vi "Add Extensions to Available Jobs.vi"(8 "error in (no error)":errorcluster) -> (0 "error out":errorcluster)   [LabVIEW 2014]
uses:
  <vilib>/Utility/traverseref.llb/TRef TravTarget.ctl
  <vilib>/Utility/miscctls.llb/LVPointTypeDef.ctl
  <vilib>/Utility/traverseref.llb/VI Scripting - Traverse.lvlib
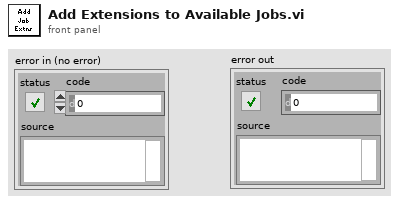
[diagram p1: front panel]
types:
  T1 = typedef "TRef TravTarget.ctl" = enum16{"FP", "BD", "Other"}
  T2 = typedef "LVPointTypeDef.ctl" = cluster{"Horizontal":i16, "Vertical":i16}
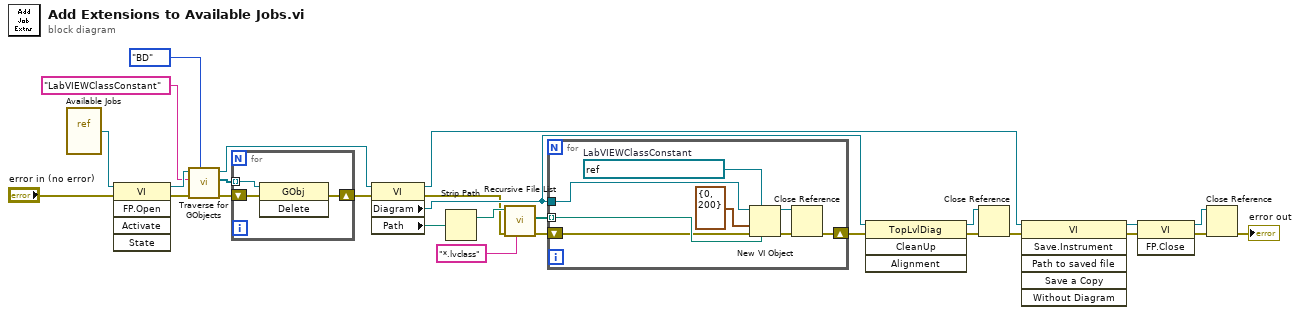
[diagram p0: block diagram]
diagram:
  n1 = vi-ref "Available Jobs.vi"() -> (w27:refnum<vi>)
  n2 = invoke class="VI" method="FP.Open"(reference=w27, error in="error in (no error)") -> (reference out=w8:refnum<vi>, error out=w6:errorcluster)  [unwired: 3 in, 3 out]
  n3 = call <vilib>:"Traverse for GObjects.vi"("Traverse Target"=TRef_TravTarget."BD", "error in (no error)"=w6, "Class Name"="LabVIEWClassConstant", "VI Refnum"=w8) -> ("error out"=w4:errorcluster, "References"=w3:refnum<vi>[], "dup VI Refnum"=w2:refnum<vi>)  [unwired: 4 in, 1 out]
  n4 = for {
    shift-right: [w28] -> w1
    shift-left: w4 -> [w29]
    tunnel: w3 -> [w30] mode=indexing
    n5 = invoke class="GObj" method="Delete"(reference=w30, error in=w29) -> (error out=w28:errorcluster)  [unwired: 1 in, 2 out]
  }
  n6 = property class="VI"(reference=w2, error in=w1) -> (reference out=w15:refnum<vi>, error out=w20:errorcluster, "Diagram"=w22:refnum<vi>, "Path"=w26:path)
  n7 = Strip Path(path=w26) -> (stripped path=w25:path)  [unwired: 1 out]
  n8 = call <vilib>:"Recursive File List.vi"("pattern"="*.lvclass", "error in (no error)"=w20, "Folder Path"=w25) -> ("error out"=w19:errorcluster, "All Files in Dir"=w23:path[])  [unwired: 4 in, 3 out]
  n9 = for {
    tunnel: w22 -> [w38]
    tunnel: w23 -> [w35] mode=indexing
    shift-right: [w31] -> w21
    shift-left: w19 -> [w34]
    w37 = refnum<vi> refnum  # LabVIEWClassConstant
    n10 = New VI Object(vi object class=w37, owner refnum=w38, position/next to=T2 {"Horizontal"=0, "Vertical"=200} ("location"), 6:w35, 8:w34) -> (object refnum=w32:refnum<vi>, 0:w33:errorcluster)  [unwired: 3 in]
    n11 = Close Reference(reference=w32, error in (no error)=w33) -> (error out=w31:errorcluster)
  }
  n12 = invoke class="TopLvlDiag" method="CleanUp"(reference=w22, error in=w21) -> (reference out=w17:refnum<vi>, error out=w18:errorcluster)  [unwired: 2 in, 2 out]
  n13 = Close Reference(reference=w17, error in (no error)=w18) -> (error out=w16:errorcluster)
  n14 = invoke class="VI" method="Save.Instrument"(reference=w15, error in=w16) -> (reference out=w14:refnum<vi>, error out=w13:errorcluster)  [unwired: 4 in, 4 out]
  n15 = invoke class="VI" method="FP.Close"(reference=w14, error in=w13) -> (reference out=w11:refnum<vi>, error out=w12:errorcluster)  [unwired: 1 in, 1 out]
  n16 = Close Reference(reference=w11, error in (no error)=w12) -> (error out=→"error out":errorcluster)
